vi "wait.vi"(1 "State to wait for":i32, 2 "Waiting Loop ID":i32, 3 "time (ms)":i32, 4 "Current Loop ID":i32) -> (0 "Done?":bool)   [LabVIEW 2011]
doc: "This VI allows you to wait for a specified amount of time before advancing, or for a different subsystem to reach a different state. Useful in autonomous applications."
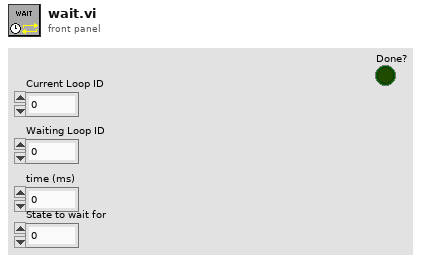
[diagram p1: front panel]
types:
  T1 = typedef "subStates.ctl" = enum16{"null", "wait", "driver control", "auto", "manual override", "autoDrive", "hold position", "rotate", "end"}
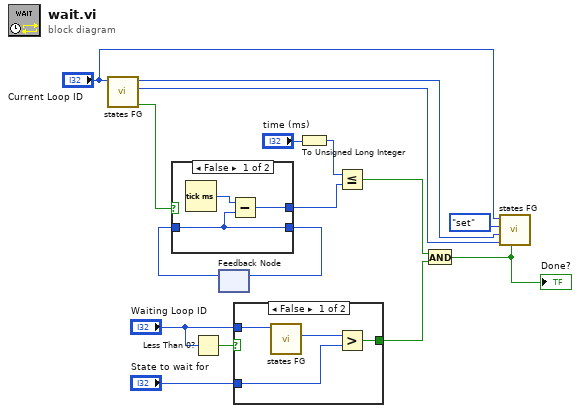
[diagram p0: block diagram]
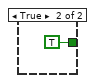
[diagram p2: hidden frame]
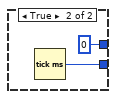
[diagram p3: hidden frame]
diagram:
  n1 = call "states FG.vi"("Loop ID"="Current Loop ID") -> ("first call?"=w16:bool, "state # out"=w5:i32, "subState out"=w6:T1)  [unwired: 7 in, 1 out]
  n2 = Less Than 0?(x="Waiting Loop ID") -> (x < 0?=w1:bool)
  n3 = feedback #1() -> (w14:u32)  [unwired: 1 in]
  n4 = case shown="False" w16 {
    tunnel: [w18 w21] -> w15
    tunnel: w14 -> [w18 _]
    tunnel: [w17 u32 0] -> w13
    frame False {
      n5 = Tick Count (ms)() -> (millisecond timer value=w19:u32)
      n6 = Subtract(x=w19, y=w18) -> (x-y=w17:u32)
    }
    frame True {
      n7 = Tick Count (ms)() -> (millisecond timer value=w21:u32)
    }
  }
  n8 = feedback-in #1(w15) -> ()
  n9 = case shown="False" w1 {
    tunnel: "Waiting Loop ID" -> [w25 _]
    tunnel: "State to wait for" -> [w24 _]
    tunnel: [w23 TRUE] -> w10
    frame False {
      n10 = call "states FG.vi"("Loop ID"=w25) -> ("state # out"=w22:i32)  [unwired: 7 in, 3 out]
      n11 = Greater?(x=w22, y=w24) -> (0:w23:bool)
    }
    frame True {
    }
  }
  n12 = To Unsigned Long Integer(number="time (ms)") -> (unsigned 32bit integer=w3:u32)
  n13 = Less Or Equal?(x=w3, y=w13) -> (x <= y?=w11:bool)
  n14 = And(x=w11, y=w10) -> (x .and. y?=w9:bool)
  "Done?" <- w9
  n15 = call "states FG.vi"("exit in"=w9, "state # in"=w5, "subState in"=w6, "menu (get)"=enum16{"set", "get"}."set", "Loop ID"="Current Loop ID") -> ()  [unwired: 3 in, 4 out]
